vi "Intake Global.vi"() -> ()   [LabVIEW 2019]
panel:
  in  "Intake Speed":dbl
  out "Intake Piston":bool
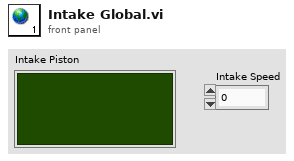
[diagram p1: front panel]
diagram:
